vi "Read Update period.vi"(8 "error in (no error)":errorcluster, 11 "Instrument Recorder in":refnum<class "Instrument Recorder.lvclass">) -> (0 "error out":errorcluster, 2 "Update period":i32=10, 3 "Instrument Recorder out":refnum<class "Instrument Recorder.lvclass">)   [LabVIEW 2015, in "Instrument Recorder.lvclass"]
uses:
  Instrument Recorder.lvclass
  Instrument Recorder.lvclass/Instrument Recorder.ctl
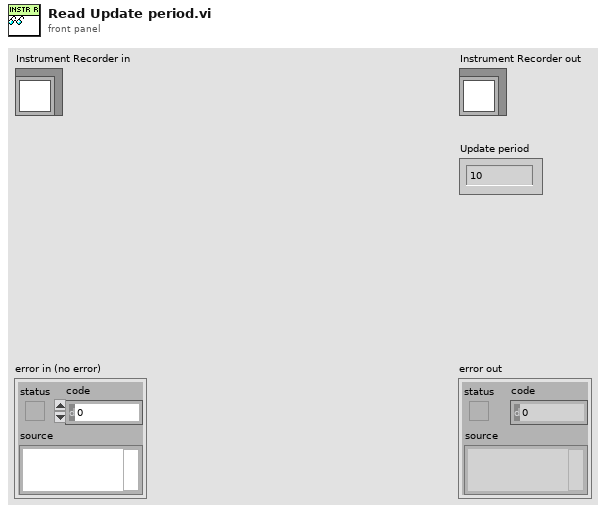
[diagram p1: front panel]
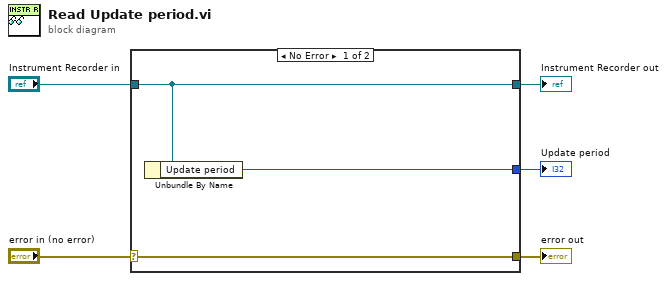
[diagram p0: block diagram]
diagram:
  n1 = case shown="No Error" "error in (no error)" {
    selector: "error in (no error)" -> [w8 w9]
    tunnel: [w8 w9] -> w4
    tunnel: [w7 w10] -> w2
    tunnel: "Instrument Recorder in" -> [w7 w10]
    tunnel: [w6 _] -> w1
    frame No Error {
      n2 = Unbundle By Name(w7) -> ("Update period"=w6:i32)
    }
    frame Error {
    }
  }
  "error out" <- w4
  "Instrument Recorder out" <- w2
  "Update period" <- w1
